vi "mean_std_var_Complex.vi"(8 "Weighting (Sample)":enum16{"Sample", "Population", ""}(ring), 11 "Input Array":cdb[](array[numeric])=[2.0-4.0i, 10.0+1.0i, -7.0-7.0i, 2.0+1.0i]) -> (1 "variance":dbl=63.833333333333336, 2 "standard deviation":dbl=7.989576542804589, 3 "mean":cdb=1.75-2.25i)   [LabVIEW 2021]
panel:
  # "I wrote this vi because LabView's built in version doesn't allow for complex inputs. \nThis gives the same value as matlab's std and var commands (using \"Sample\")."
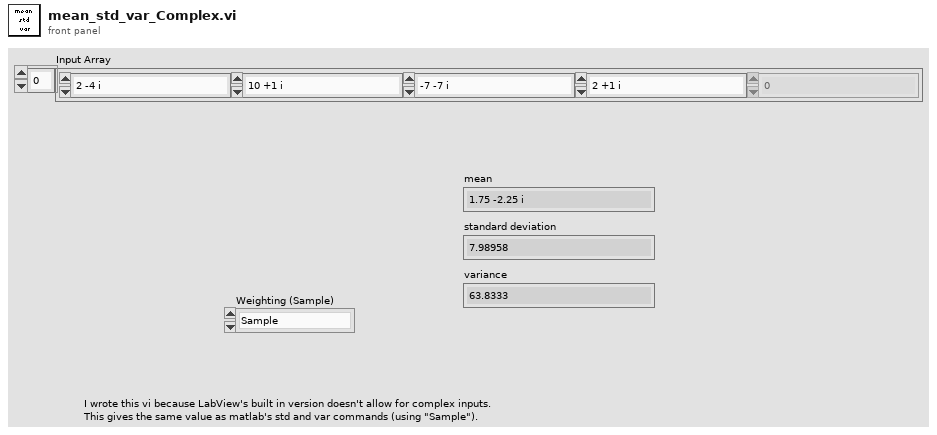
[diagram p1: front panel]
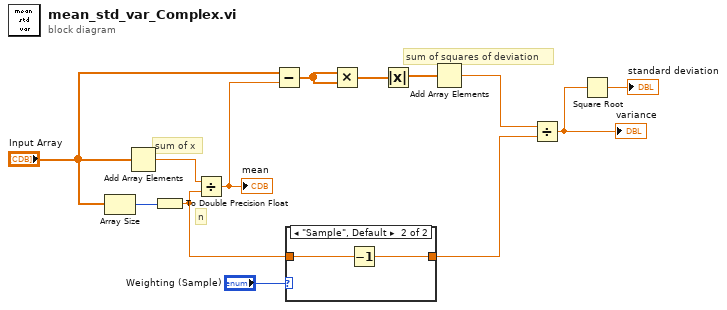
[diagram p0: block diagram]
diagram:
  # "n"
  # "sum of x"
  # "sum of squares of deviation"
  n1 = Array Size(array="Input Array") -> (size(s)=w12:i32)
  n2 = Add Array Elements(numeric array="Input Array") -> (sum=w13:cdb)
  n3 = To Double Precision Float(number=w12) -> (double precision float=w6:dbl)
  n4 = Divide(x=w13, y=w6) -> (x/y=w11:cdb)
  "mean" <- w11
  n5 = Subtract(x="Input Array", y=w11) -> (x-y=w9:cdb[])
  n6 = case shown="\"Sample\", Default" "Weighting (Sample)" {
    tunnel: w6 -> [w14 w16]
    tunnel: [w14 w15] -> w5
    frame "Population" {
    }
    frame "Sample", Default {
      n7 = Decrement(x=w16) -> (x-1=w15:dbl)
    }
  }
  n8 = Multiply(x=w9, y=w9) -> (x*y=w2:cdb[])
  n9 = Absolute Value(x=w2) -> (abs(x)=w1:dbl[])
  n10 = Add Array Elements(numeric array=w1) -> (sum=w8:dbl)
  n11 = Divide(x=w8, y=w5) -> (x/y=w4:dbl)
  "variance" <- w4
  n12 = Square Root(x=w4) -> (sqrt(x)=→"standard deviation":dbl)
